vi "Sub04_Tracing.vi"(8 "CommandInfo":T1={"RedBall"={"Min"={"G"=0, "B"=0, "R"=160}, "Max"={"G"=160, "B"=160, "R"=255}}, "YellowBall"={"Min"={"G"=140, "B"=0, "R"=140}, "Max"={"G"=255, "B"=175, "R"=255}}, "WhiteBall"={"Min"={"G"=100, "B"=100, "R"=100}, "Max"={"G"=255, "B"=255, "R"=255}}, "BallDiameter"=11, "BackGround"={"Min"={"G"=91, "B"=202, "R"=39}, "Max"={"G"=116, "B"=255, "R"=62}}, "Border"={"Min"={"G"=0, "B"=121, "R"=0}, "Max"={"G"=42, "B"=126, "R"=14}}}, 10 "new picture in":picture, 11 "Array":T2(array[cluster])) -> (3 "new picture out":picture)   [LabVIEW 2019]
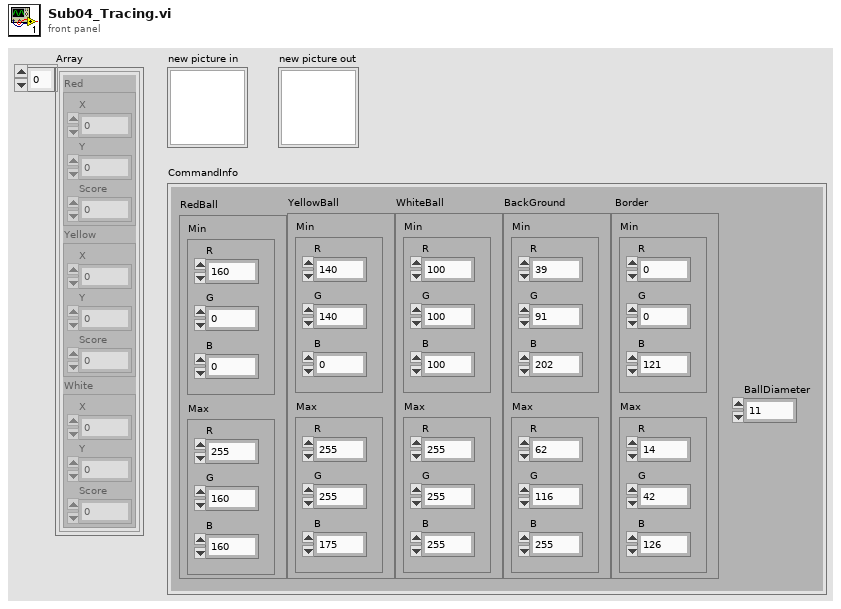
[diagram p1: front panel]
types:
  T1 = cluster{"RedBall":cluster{"Min":cluster{"G":u32, "B":u32, "R":u32}, "Max":cluster{"G":u32, "B":u32, "R":u32}}, "YellowBall":cluster{"Min":cluster{"G":u32, "B":u32, "R":u32}, "Max":cluster{"G":u32, "B":u32, "R":u32}}, "WhiteBall":cluster{"Min":cluster{"G":u32, "B":u32, "R":u32}, "Max":cluster{"G":u32, "B":u32, "R":u32}}, "BallDiameter":u32, "BackGround":cluster{"Min":cluster{"G":u32, "B":u32, "R":u32}, "Max":cluster{"G":u32, "B":u32, "R":u32}}, "Border":cluster{"Min":cluster{"G":u32, "B":u32, "R":u32}, "Max":cluster{"G":u32, "B":u32, "R":u32}}}
  T2 = cluster{"Red":cluster{"X":u32, "Y":u32, "Score":u32}, "Yellow":cluster{"X":u32, "Y":u32, "Score":u32}, "White":cluster{"X":u32, "Y":u32, "Score":u32}}[]
  T3 = cluster{"Min":cluster{"G":u32, "B":u32, "R":u32}, "Max":cluster{"G":u32, "B":u32, "R":u32}}
  T4 = cluster{"Red":cluster{"X":u32, "Y":u32, "Score":u32}, "Yellow":cluster{"X":u32, "Y":u32, "Score":u32}, "White":cluster{"X":u32, "Y":u32, "Score":u32}}
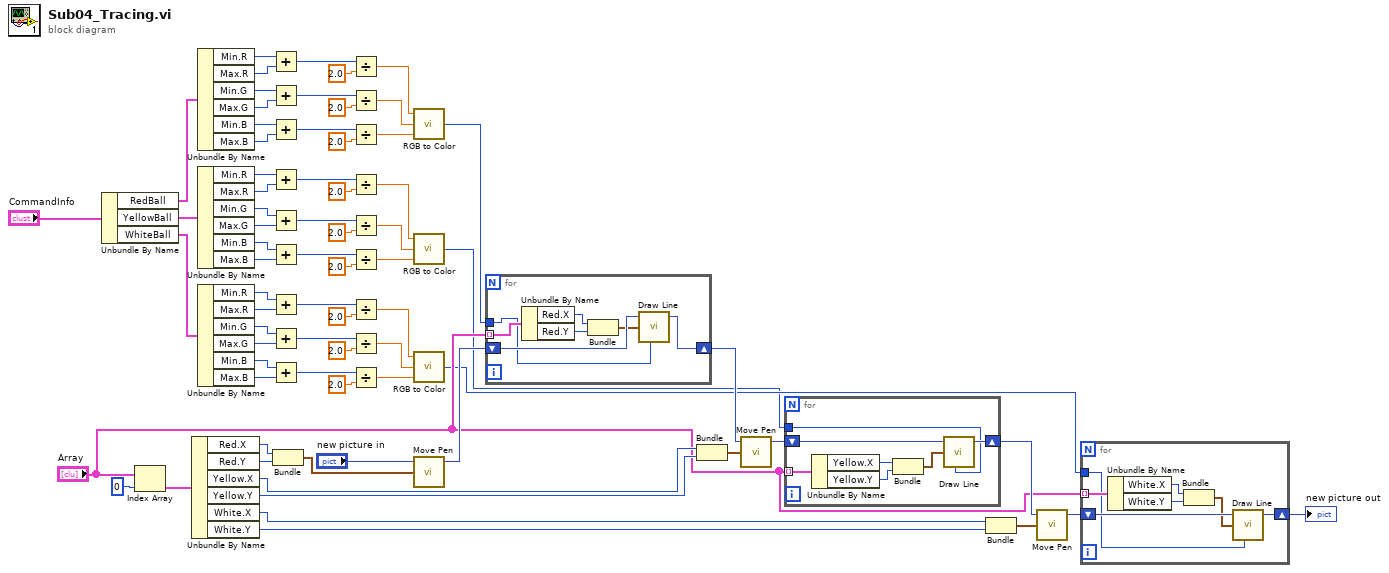
[diagram p0: block diagram]
diagram:
  n1 = Unbundle By Name("CommandInfo") -> ("RedBall"=w2:T3, "YellowBall"=w19:T3, "WhiteBall"=w51:T3)
  n2 = Index Array(array="Array", index=0) -> (element=w68:T4)
  n3 = Unbundle By Name(w68) -> ("Red.X"=w69:u32, "Red.Y"=w70:u32, "Yellow.X"=w64:u32, "Yellow.Y"=w63:u32, "White.X"=w62:u32, "White.Y"=w61:u32)
  n4 = Unbundle By Name(w2) -> ("Min.R"=w14:u32, "Max.R"=w13:u32, "Min.G"=w9:u32, "Max.G"=w8:u32, "Min.B"=w4:u32, "Max.B"=w3:u32)
  n5 = Unbundle By Name(w19) -> ("Min.R"=w31:u32, "Max.R"=w30:u32, "Min.G"=w26:u32, "Max.G"=w25:u32, "Min.B"=w21:u32, "Max.B"=w20:u32)
  n6 = Unbundle By Name(w51) -> ("Min.R"=w46:u32, "Max.R"=w45:u32, "Min.G"=w41:u32, "Max.G"=w40:u32, "Min.B"=w36:u32, "Max.B"=w35:u32)
  n7 = Add(x=w14, y=w13) -> (x+y=w17:u32)
  n8 = Add(x=w9, y=w8) -> (x+y=w12:u32)
  n9 = Add(x=w4, y=w3) -> (x+y=w7:u32)
  n10 = Add(x=w31, y=w30) -> (x+y=w34:u32)
  n11 = Add(x=w26, y=w25) -> (x+y=w29:u32)
  n12 = Add(x=w21, y=w20) -> (x+y=w24:u32)
  n13 = Add(x=w46, y=w45) -> (x+y=w49:u32)
  n14 = Add(x=w41, y=w40) -> (x+y=w44:u32)
  n15 = Add(x=w36, y=w35) -> (x+y=w39:u32)
  n16 = Bundle("X"=w69, "Y"=w70) -> (w71:cluster{"X":u32, "Y":u32})  [unwired: 1 in]
  n17 = Divide(x=w17, y=2.0) -> (x/y=w15:dbl)
  n18 = Divide(x=w12, y=2.0) -> (x/y=w10:dbl)
  n19 = Divide(x=w7, y=2.0) -> (x/y=w5:dbl)
  n20 = Divide(x=w34, y=2.0) -> (x/y=w32:dbl)
  n21 = Divide(x=w29, y=2.0) -> (x/y=w27:dbl)
  n22 = Divide(x=w24, y=2.0) -> (x/y=w22:dbl)
  n23 = Divide(x=w49, y=2.0) -> (x/y=w47:dbl)
  n24 = Divide(x=w44, y=2.0) -> (x/y=w42:dbl)
  n25 = Divide(x=w39, y=2.0) -> (x/y=w37:dbl)
  n26 = call <vilib>:"RGB to Color.vi"("B"=w5, "G"=w10, "R"=w15) -> ("Color"=w1:u32)
  n27 = call <vilib>:"RGB to Color.vi"("B"=w22, "G"=w27, "R"=w32) -> ("Color"=w18:u32)
  n28 = call <vilib>:"RGB to Color.vi"("B"=w37, "G"=w42, "R"=w47) -> ("Color"=w50:u32)
  n29 = call <vilib>:"Move Pen.vi"("new position"=w71, "picture"="new picture in") -> ("new picture"=w66:picture)  [unwired: 3 in]
  n30 = for {
    tunnel: "Array" -> [w76] mode=indexing
    shift-right: [w77] -> w58
    shift-left: w66 -> [w78]
    tunnel: w1 -> [w72]
    n31 = Unbundle By Name(w76) -> ("Red.X"=w75:u32, "Red.Y"=w74:u32)
    n32 = Bundle("X"=w75, "Y"=w74) -> (w73:cluster{"X":u32, "Y":u32})  [unwired: 1 in]
    n33 = call <vilib>:"Draw Line.vi"("picture"=w78, "end point"=w73, "color(black)"=w72) -> ("new picture"=w77:picture)  [unwired: 6 in]
  }
  n34 = Bundle("X"=w64, "Y"=w63) -> (w60:cluster{"X":u32, "Y":u32})  [unwired: 1 in]
  n35 = call <vilib>:"Move Pen.vi"("new position"=w60, "picture"=w58) -> ("new picture"=w57:picture)  [unwired: 3 in]
  n36 = for {
    tunnel: "Array" -> [w83] mode=indexing
    shift-right: [w84] -> w55
    shift-left: w57 -> [w85]
    tunnel: w18 -> [w79]
    n37 = Unbundle By Name(w83) -> ("Yellow.X"=w82:u32, "Yellow.Y"=w81:u32)
    n38 = Bundle("X"=w82, "Y"=w81) -> (w80:cluster{"X":u32, "Y":u32})  [unwired: 1 in]
    n39 = call <vilib>:"Draw Line.vi"("picture"=w85, "end point"=w80, "color(black)"=w79) -> ("new picture"=w84:picture)  [unwired: 6 in]
  }
  n40 = Bundle("X"=w62, "Y"=w61) -> (w59:cluster{"X":u32, "Y":u32})  [unwired: 1 in]
  n41 = call <vilib>:"Move Pen.vi"("new position"=w59, "picture"=w55) -> ("new picture"=w56:picture)  [unwired: 3 in]
  n42 = for {
    tunnel: "Array" -> [w90] mode=indexing
    shift-right: [w91] -> w54
    shift-left: w56 -> [w92]
    tunnel: w50 -> [w86]
    n43 = Unbundle By Name(w90) -> ("White.X"=w89:u32, "White.Y"=w88:u32)
    n44 = Bundle("X"=w89, "Y"=w88) -> (w87:cluster{"X":u32, "Y":u32})  [unwired: 1 in]
    n45 = call <vilib>:"Draw Line.vi"("picture"=w92, "end point"=w87, "color(black)"=w86) -> ("new picture"=w91:picture)  [unwired: 6 in]
  }
  "new picture out" <- w54
